vi "List Launchpads.vi"(8 "error in":errorcluster) -> (0 "error out":errorcluster, 2 "Devices":string[](array[string]), 3 "Com Port":i32[](array[numeric]))   [LabVIEW 2014]
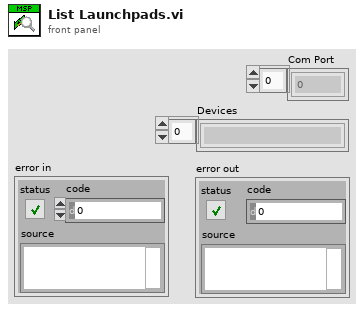
[diagram p1: front panel]
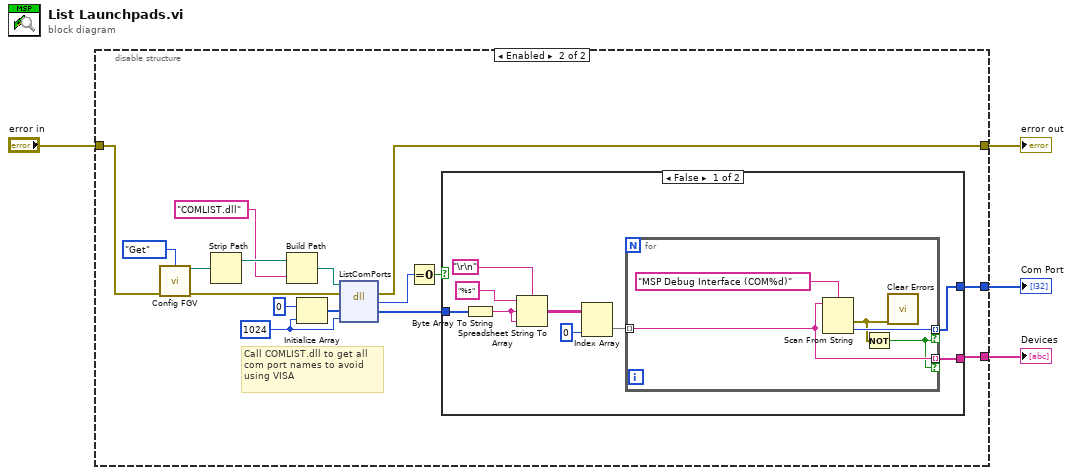
[diagram p0: block diagram]
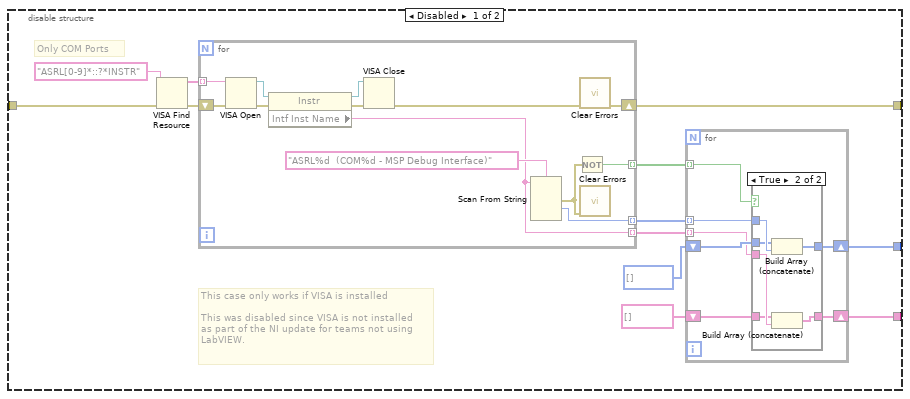
[diagram p2: hidden frame]
diagram:
  n1 = disable-structure shown="Enabled" {
    disable-tunnel: "error in" -> [w14 w51]
    disable-tunnel: [w13 w54] -> w3
    disable-tunnel: [w7 w53] -> w2
    disable-tunnel: [w6 w52] -> w1
    frame Disabled {
      # "This case only works if VISA is installed\n\nThis was disabled since VISA is not installed \nas part of the NI update for teams not using\nLabVIEW."
      # "Only COM Ports"
      n2 = VISA Find Resource(8:w14, 11:"ASRL[0-9]*::?*INSTR" ("expression (\"?*\")")) -> (0:w15:errorcluster, 3:w16:string[])  [unwired: 1 in, 1 out]
      n3 = for {
        tunnel: w16 -> [w41] mode=indexing
        shift-right: [w37] -> w13
        shift-left: w15 -> [w40]
        tunnel: [w35] -> w10 mode=indexing
        tunnel: [w34] -> w11 mode=indexing
        tunnel: [w32] -> w12 mode=indexing
        n4 = VISA Open(error in (no error)=w40, VISA resource name=w41) -> (VISA resource name=w43:refnum<visa-resource-name>, error out=w42:errorcluster)  [unwired: 3 in]
        n5 = property class="Instr"(reference=w43, error in=w42) -> (reference out=w44:refnum<visa-resource-name>, error out=w39:errorcluster, "Intf Inst Name"=w34:string)
        n6 = VISA Close(VISA resource name=w44, error in (no error)=w39) -> (error out=w38:errorcluster)
        n7 = Scan From String(format string="ASRL%d  (COM%d - MSP Debug Interface)", input string=w34) -> (error out=w33:errorcluster, output 1=w35:i32)  [unwired: 5 in, 2 out]
        n8 = Not(x=w33) -> (.not. x?=w32:bool)
        n9 = call <vilib>:"Clear Errors.vi"("error in (no error)"=w38) -> ("error out"=w37:errorcluster)  [unwired: 5 in, 1 out]
        n10 = call <vilib>:"Clear Errors.vi"("error in (no error)"=w33) -> ()  [unwired: 5 in, 2 out]
      }
      n11 = for {
        tunnel: w12 -> [w23] mode=indexing
        tunnel: w11 -> [w19] mode=indexing
        tunnel: w10 -> [w22] mode=indexing
        shift-right: [w21] -> w6
        shift-left: i32[] [] -> [w20]
        shift-right: [w18] -> w7
        shift-left: string[] [] -> [w17]
        n12 = case shown="True" w23 {
          tunnel: w22 -> [_ w31]
          tunnel: [w25 w30] -> w21
          tunnel: w20 -> [w25 w29]
          tunnel: w19 -> [_ w28]
          tunnel: [w24 w27] -> w18
          tunnel: w17 -> [w24 w26]
          frame False {
          }
          frame True {
            n13 = Build Array (concatenate)(w29, w31) -> (w30:i32[])
            n14 = Build Array (concatenate)(w26, w28) -> (w27:string[])
          }
        }
      }
    }
    frame Enabled {
      w58 = 1024
      # "Call COMLIST.dll to get all\ncom port names to avoid\nusing VISA"
      n15 = call "Config FGV.vi"("Operation"=enum16{"Get", "Set"}."Get", "error in"=w51) -> ("Tool Path"=w48:path, "error out"=w50:errorcluster)  [unwired: 9 in, 3 out]
      n16 = Strip Path(path=w48) -> (stripped path=w47:path)  [unwired: 1 out]
      n17 = Build Path(base path=w47, name or relative path="COMLIST.dll") -> (appended path=w46:path)
      n18 = Initialize Array(u8 0, w58) -> (w59:u8[])
      n19 = dll-call lib="C:/Users/a0272913/Desktop/Gamepad Tool/Tools/mspdebug/COMLIST.dll" fn="ListComPorts"(path in=w46, error in=w50, "ComPorts"=w59, "size"=w58) -> (error out=w54:errorcluster, "return type"=w56:i32, "ComPorts"=w57:u8[])  [unwired: 2 in, 1 out]
      n20 = Equal To 0?(x=w56) -> (x = 0?=w55:bool)
      n21 = case shown="False" w55 {
        tunnel: w57 -> [w69 _]
        tunnel: [w62 _] -> w53
        tunnel: [w61 _] -> w52
        frame False {
          n22 = Byte Array To String(unsigned byte array=w69) -> (string=w68:string)
          n23 = Spreadsheet String To Array(delimiter (Tab)="\r\n", format string="%s", spreadsheet string=w68, array type (2D Dbl)=w68) -> (array=w65:string[][])
          n24 = Index Array(array=w65, index (col)=0 ("disabled index (col)")) -> (element=w63:string[])  [unwired: 1 in]
          n25 = for {
            tunnel: [w73] -> w61 mode=indexing if=w70
            tunnel: [w71] -> w62 mode=indexing if=w70
            tunnel: w63 -> [w71] mode=indexing
            n26 = Scan From String(format string="MSP Debug Interface (COM%d)", input string=w71) -> (error out=w72:errorcluster, output 1=w73:i32)  [unwired: 3 in, 2 out]
            n27 = Not(x=w72) -> (.not. x?=w70:bool)
            n28 = call <vilib>:"Clear Errors.vi"("error in (no error)"=w72) -> ()  [unwired: 5 in, 2 out]
          }
        }
        frame True {
        }
      }
    }
  }
  "error out" <- w3
  "Devices" <- w2
  "Com Port" <- w1
